vi "TrimWhiteSpaces.vi"() -> ()   [LabVIEW 2019]
panel:
  out "length 2":i32
  out "length":i32
  out "StrippedStr":string
  in  "String1":string="     Pomogranate                        "
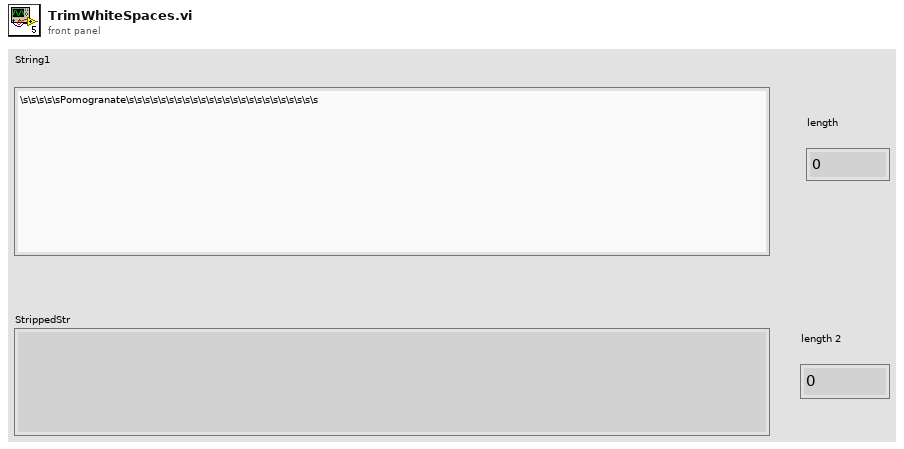
[diagram p1: front panel]
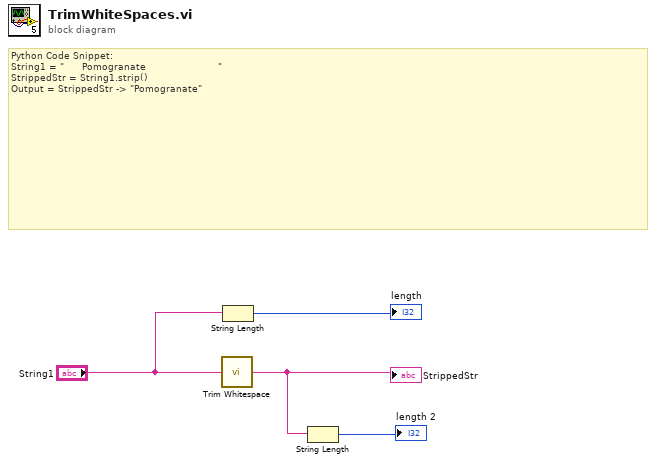
[diagram p0: block diagram]
diagram:
  # "Python Code Snippet:\nString1 = \"      Pomogranate                        \"\nStrippedStr = String1.strip()\nOutput = StrippedStr -> \"Pomogranate\""
  n1 = call <vilib>:"Trim Whitespace.vi"("string"="String1") -> ("trimmed string"=w2:string)  [unwired: 1 in]
  "StrippedStr" <- w2
  n2 = String Length(string="String1") -> (length=→"length":i32)
  n3 = String Length(string=w2) -> (length=→"length 2":i32)
